vi "Process.vi"(0 "reference in":refnum<class "Logger.lvclass">, 5 "error in":errorcluster) -> (14 "reference out":refnum<class "Logger.lvclass">, 19 "error out":errorcluster)   [LabVIEW 2023, in "Logger.lvclass"]
uses:
  Logger.lvclass
  <vilib>/HPS-17000/MStream_grpc_CyclerMeasurement.ctl
  <instrlib>/HPS-17000/HPS-17000.lvclass
  <instrlib>/HPS-17000/Internal/Read Measurement Multi.vi
  Logger.lvclass/Logger.ctl
  <vilib>/Utility/SystemLogging/NI_SystemLogging.lvlib
  <vilib>/HPS-17000/NI_BC_client.lvlib
panel:
  out "error info":errorcluster
  out "Last Command":string
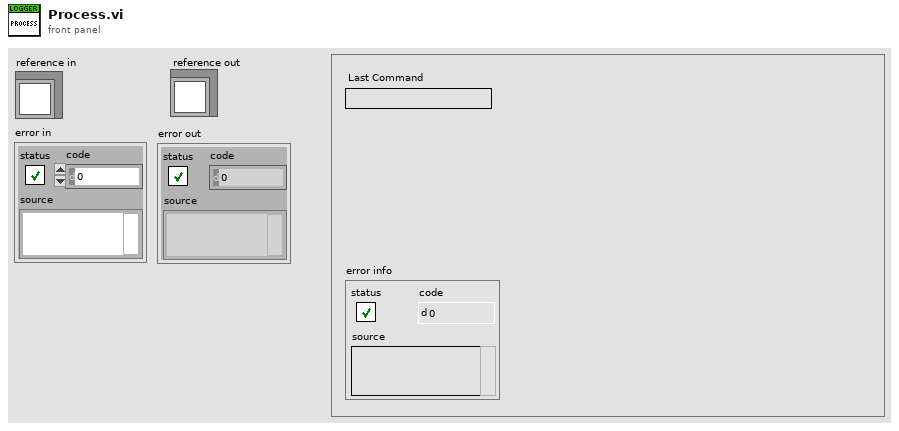
[diagram p1: front panel]
types:
  T1 = cluster{"Core":cluster{"Timeout":i32, "Events":cluster{"EventsToProcess":refnum<event-registration>}, "EventFromProcess":refnum<user-event>, "ProcessSyncQueue":refnum<queue>, "QueueFromProcess":refnum<queue>, "Command":string, "Data":variant}, "Log File Format":string, "Output Directory":path, "Log File Type":enum16{"TDMS", "CSV"}, "TDMS File":refnum<k34>, "CSV File":refnum<file>, "Logger Queue":refnum<queue>, "HPS17K Refs":refnum<class "HPS-17000.lvclass">[], "Generated Log":path, "Log Enabled":bool, "Log Created":bool}
  T2 = enum16{"open", "open or create", "create or replace", "create", "open (read-only)"}
  T3 = enum16{"open", "replace", "create", "open or create", "replace or create", "replace or create with confirmation"}
  T4 = enum32{"Invalid", "Standard", "Closed", "Hidden", "Minimized", "Maximized"}
  T5 = cluster{"EventsToProcess":refnum<event-registration>}
  T6 = typedef "Logger.lvclass/ObjectAttributes.ctl" = cluster{"Output Directory":path, "Log File Type":enum16{"TDMS", "CSV"}, "Logger Queue":refnum<queue>, "HPS17K Refs":refnum<class "HPS-17000.lvclass">[]}
  T7 = typedef "NI_BC_client.lvlib/MStream_grpc_CyclerMeasurement.ctl" = cluster{"measured_voltage":sgl, "measured_current":sgl, "setpoint_voltage":sgl, "setpoint_current":sgl, "timestamp":i64}
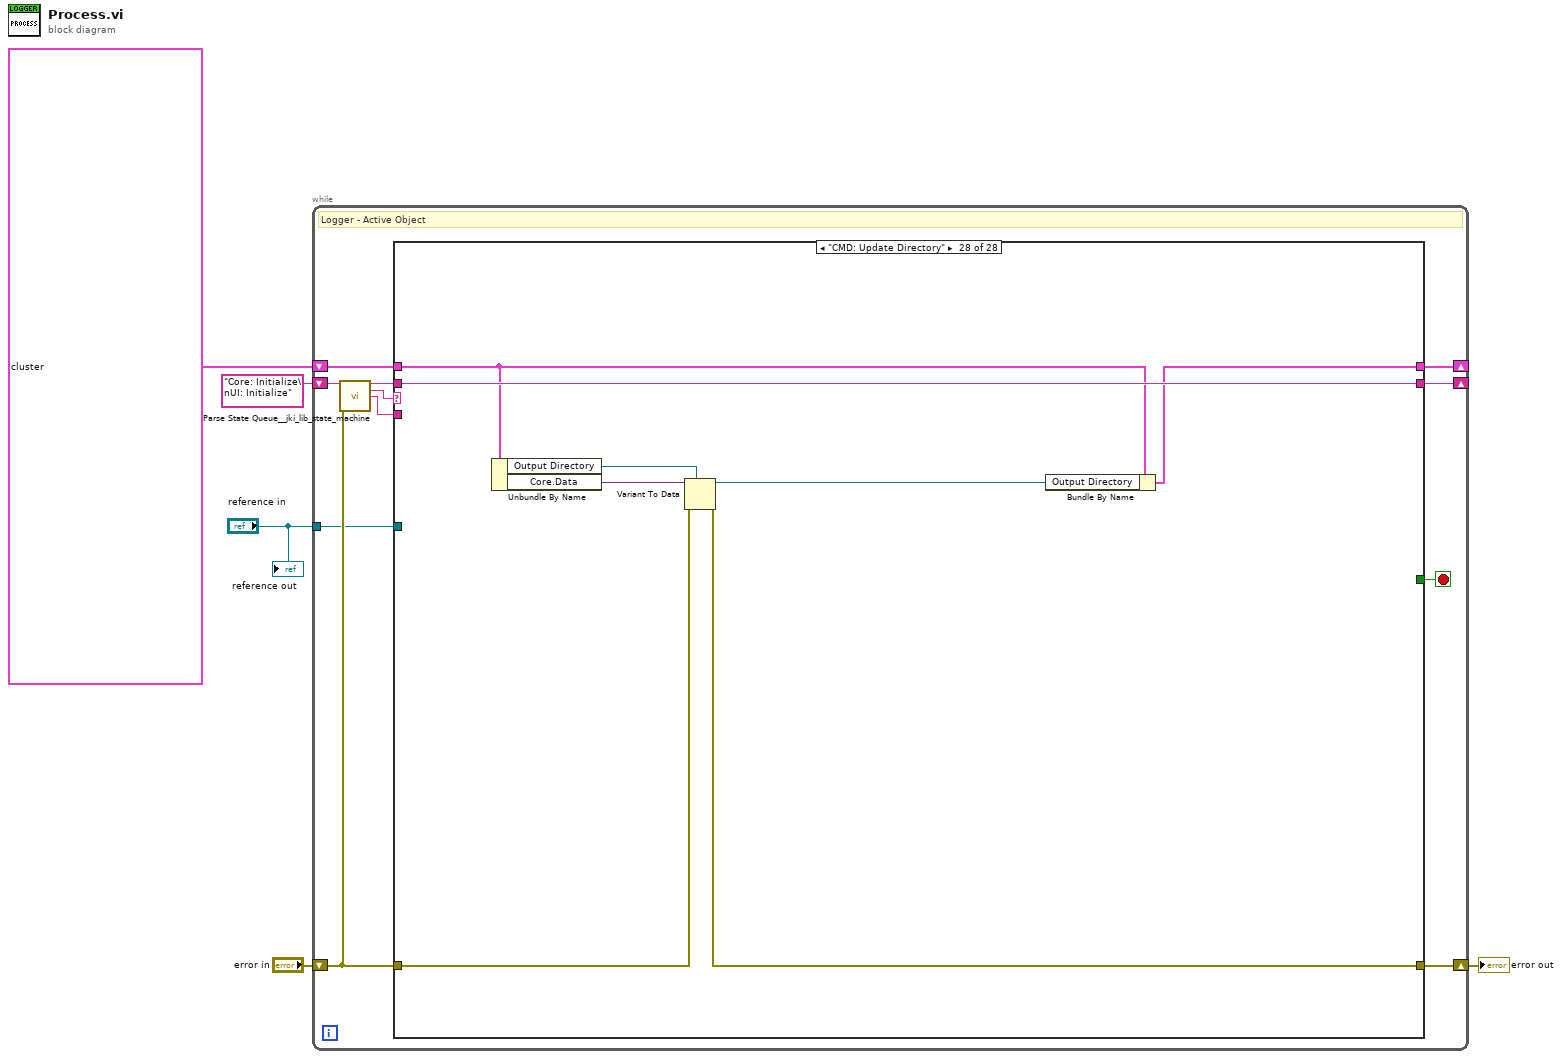
[diagram p0: block diagram]
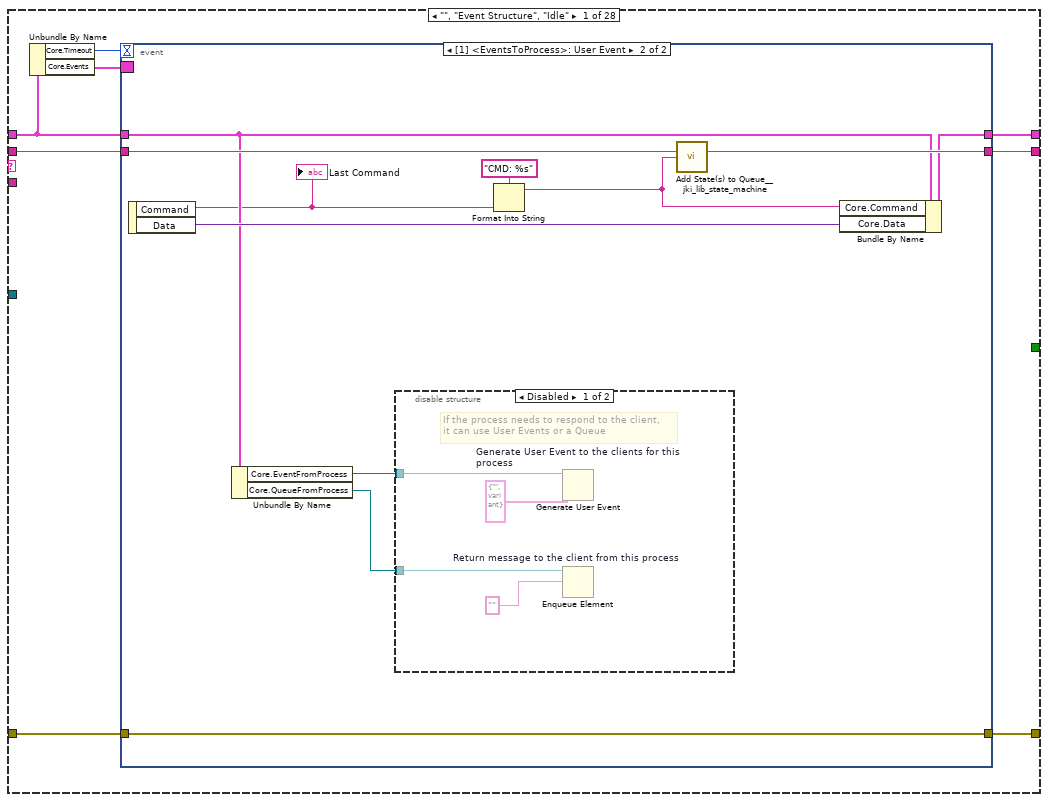
[diagram p2: hidden frame]
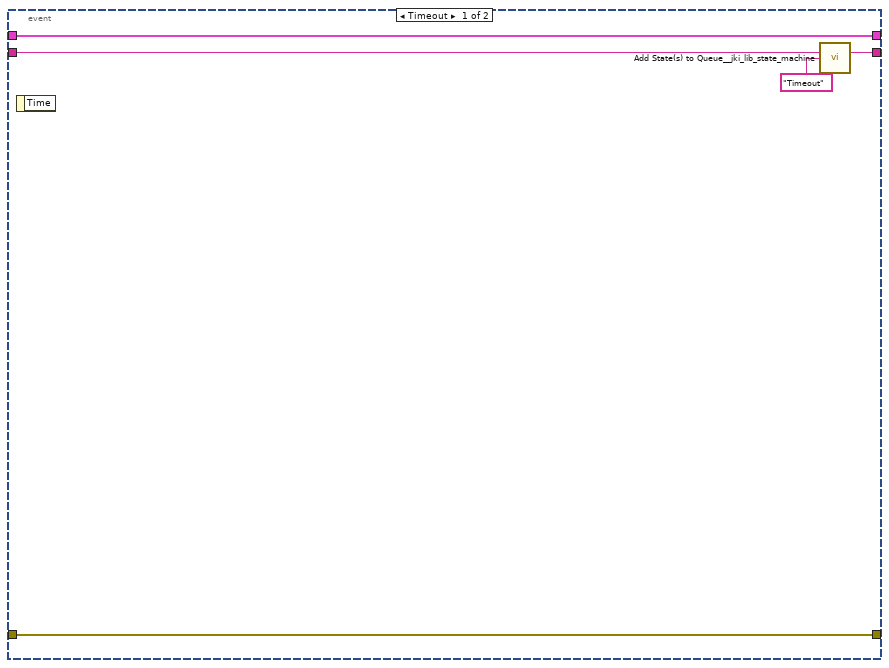
[diagram p3: hidden frame]
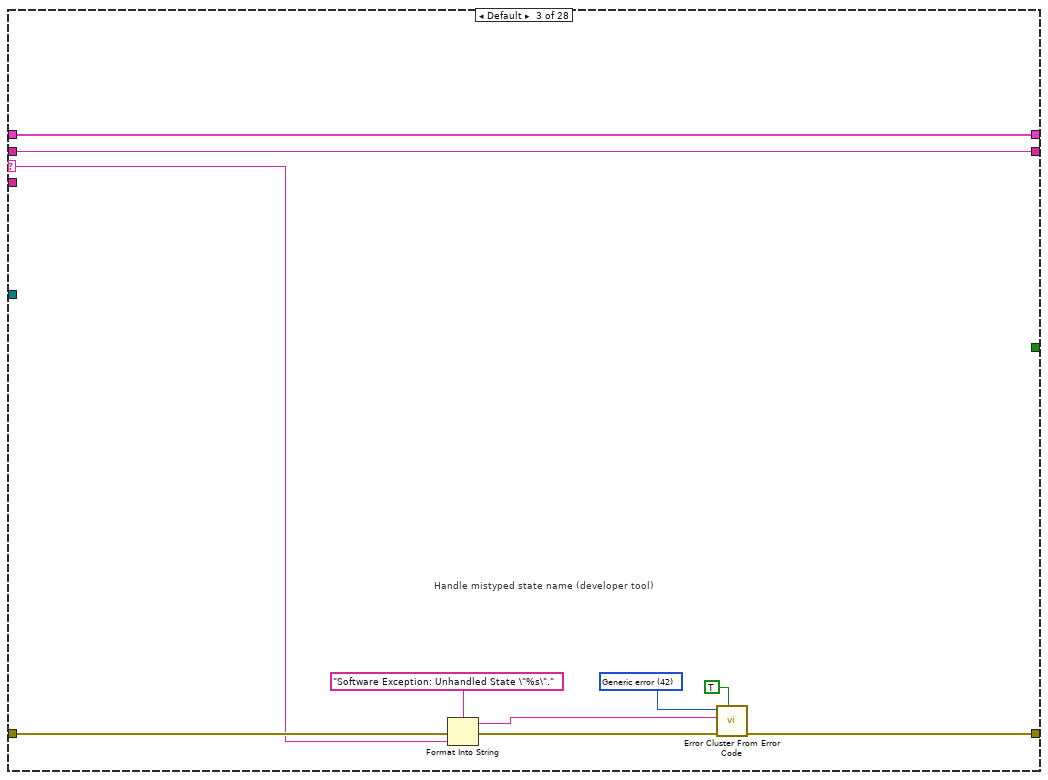
[diagram p6: hidden frame]
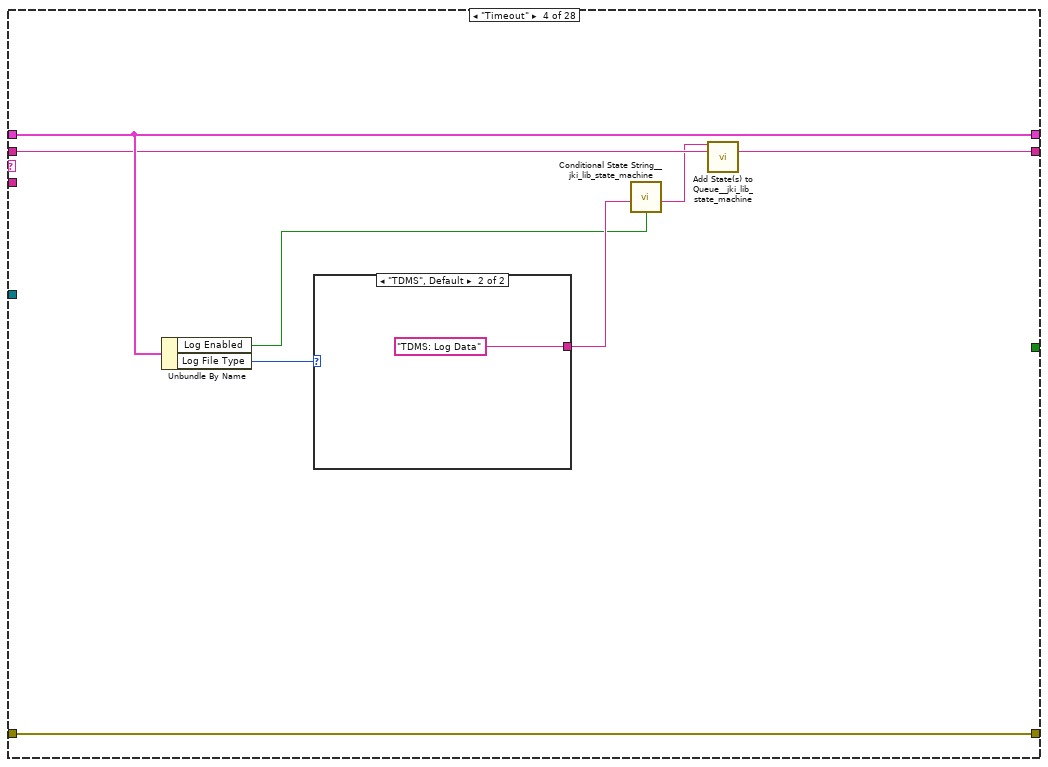
[diagram p7: hidden frame]
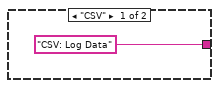
[diagram p8: hidden frame]
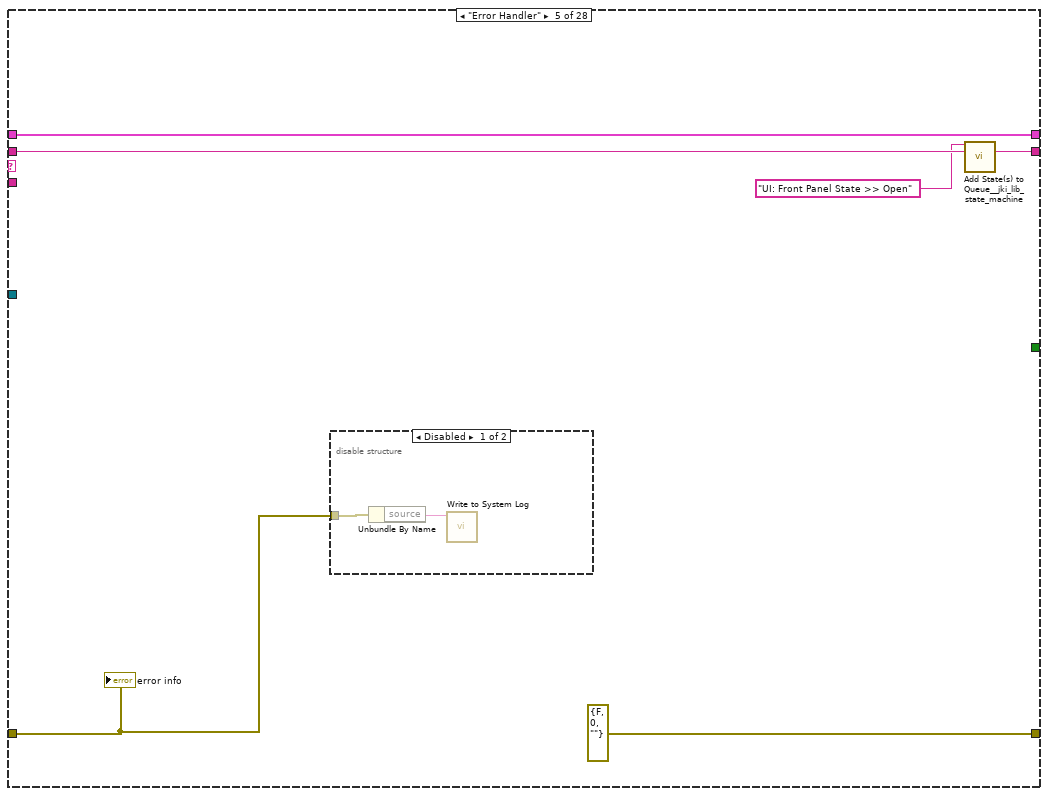
[diagram p9: hidden frame]
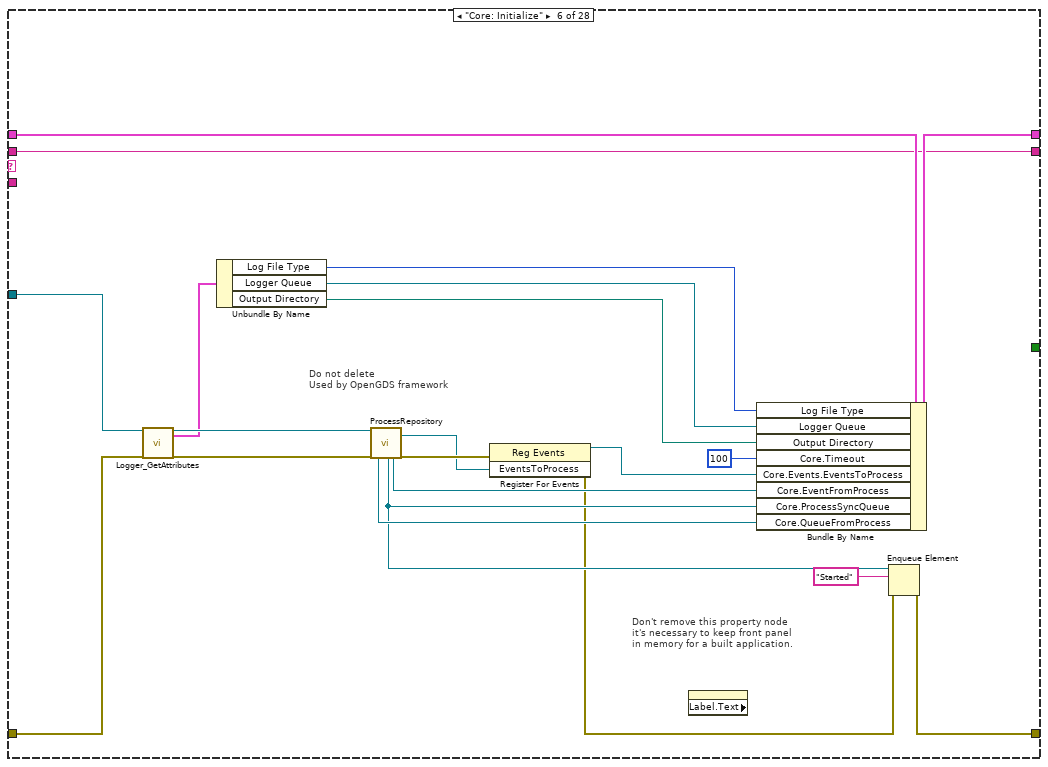
[diagram p11: hidden frame]
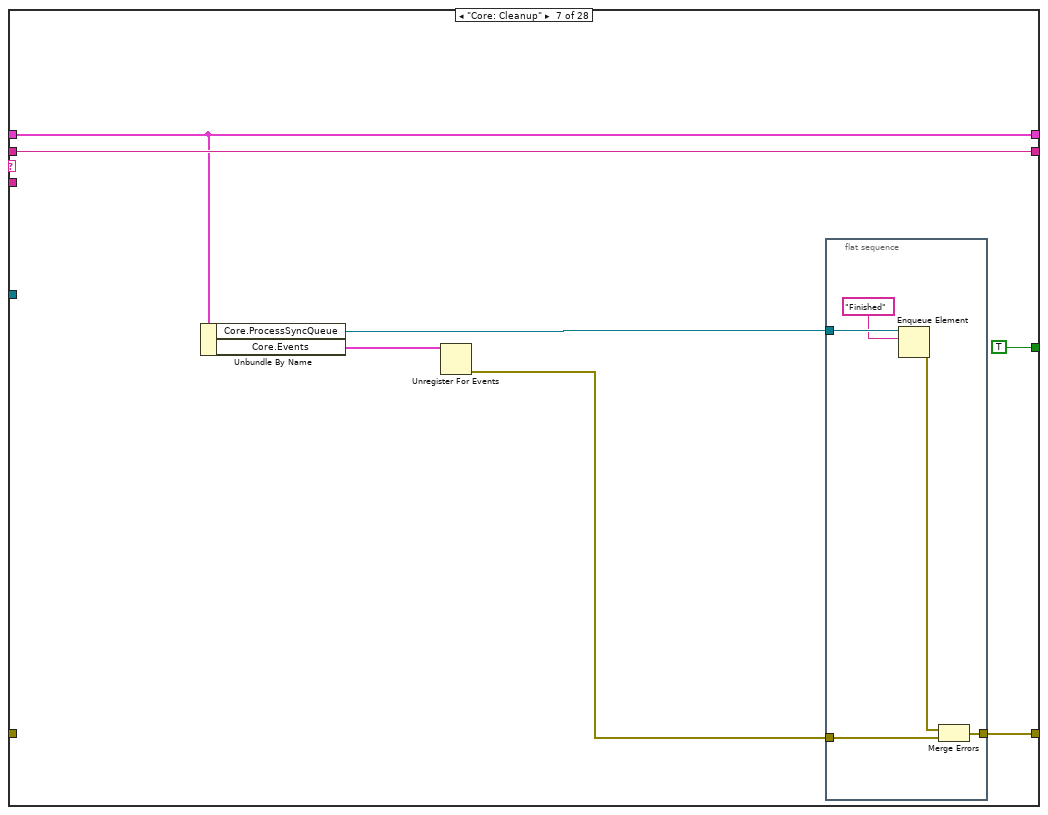
[diagram p12: hidden frame]
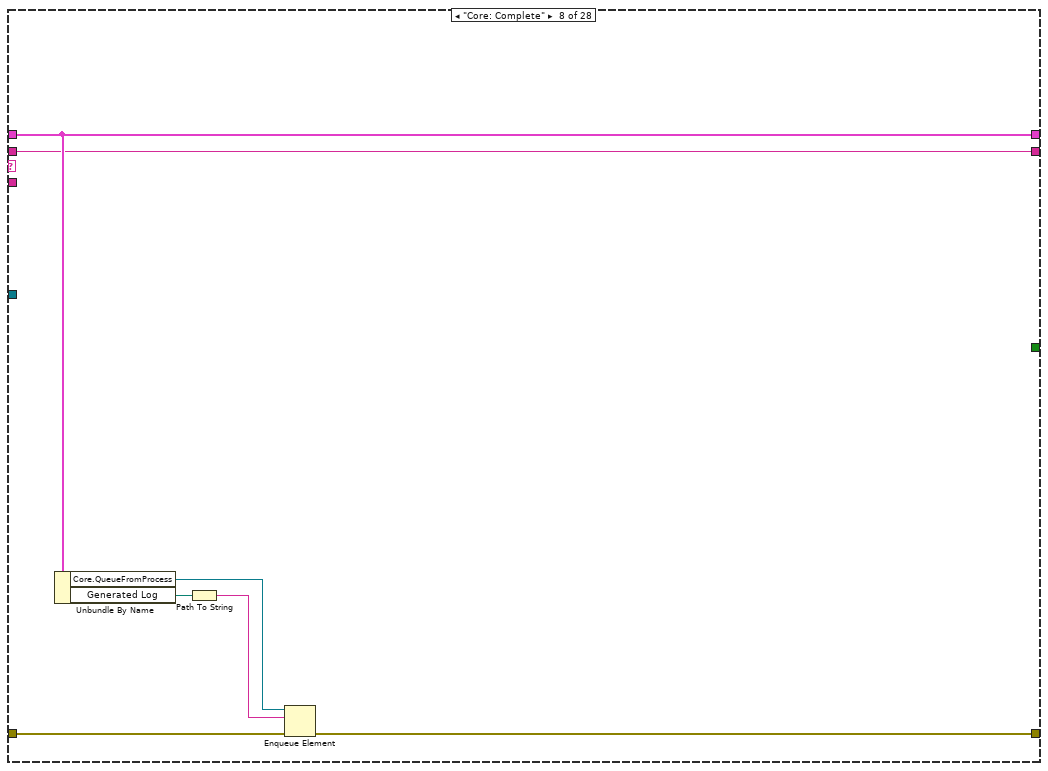
[diagram p13: hidden frame]
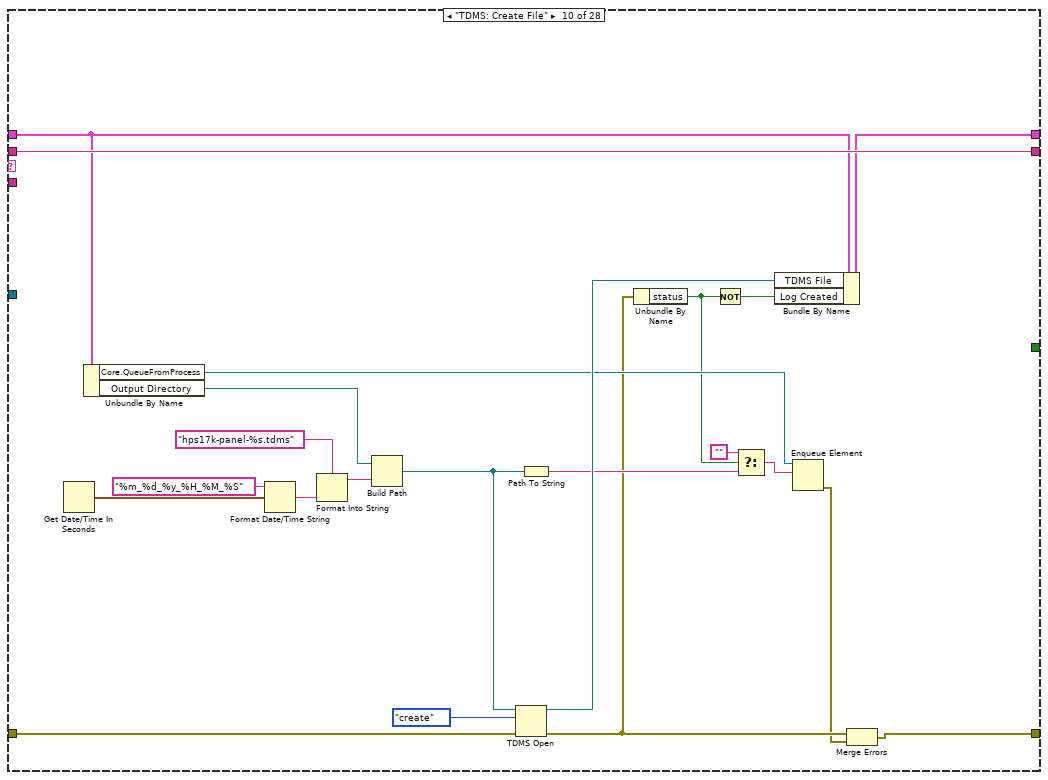
[diagram p15: hidden frame]
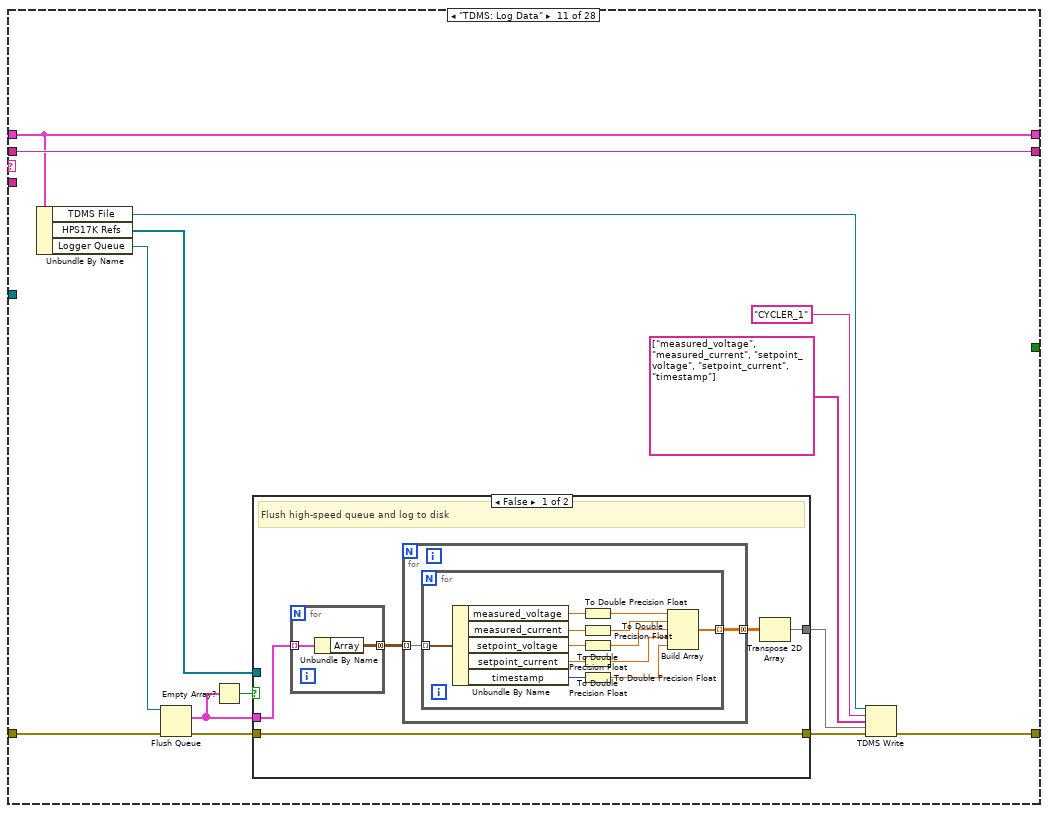
[diagram p16: hidden frame]
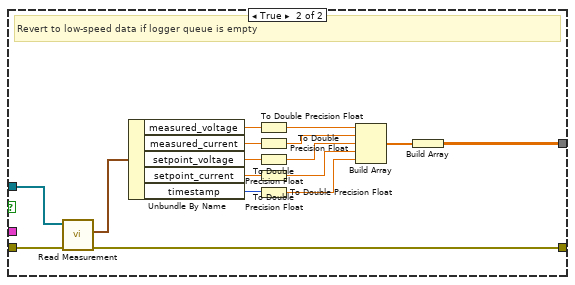
[diagram p17: hidden frame]
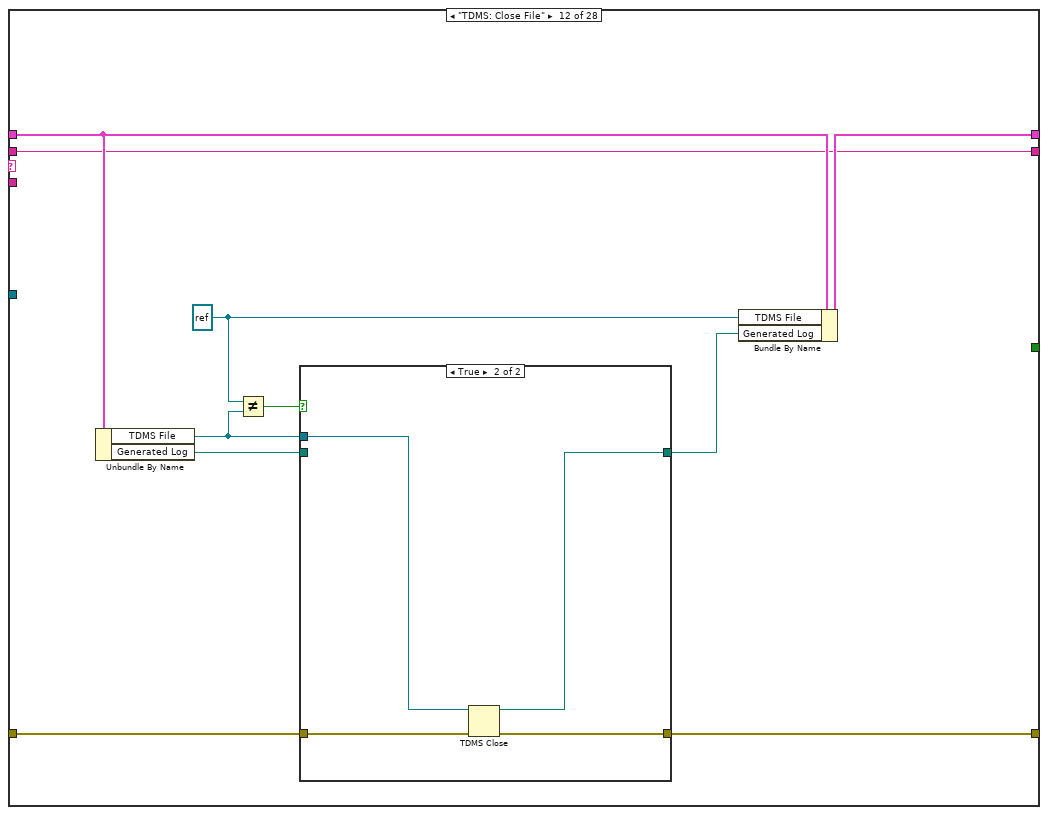
[diagram p18: hidden frame]
diagram:
  n1 = while {
    shift-right: [w15] -> w4
    shift-left: "error in" -> [w16]
    shift-right: [w8] -> _
    shift-left: "Core: Initialize\nUI: Initialize" ("States Out") -> [w11]
    shift-right: [w14] -> _
    shift-left: T1 {"Core"={"Timeout"=-1, "Events"={"EventsToProcess"=refnum}, "EventFromProcess"=refnum, "ProcessSyncQueue"=refnum, "QueueFromProcess"=refnum, "Command"="", "Data"=variant}, "Log File Format"="", "Output Directory"=path "", "Log File Type"=enum."TDMS", "TDMS File"=refnum, "CSV File"=refnum, "Logger Queue"=refnum, "HPS17K Refs"=[], "Generated Log"=path "", "Log Enabled"=FALSE, "Log Created"=FALSE} ("LocalVariables") -> [w13]
    tunnel: "reference in" -> [w6]
    stop <- w7 stop-if-true
    # "Logger - Active Object"
    n2 = call <vilib>:"Parse State Queue__jki_lib_state_machine.vi"("State Queue"=w11, "Error In (no error)"=w16) -> ("Remaining States"=w10:string, "Current State"=w12:string, "Arguments"=w9:string)  [unwired: 11 in]
    n3 = case shown="\"CMD: Update Directory\"" w12 {
      selector: w12 -> [_ _ w48 _ _ _ _ _ _ _ _ _ _ _ _ _ _ _ _ _ _ _ _ _ _ _ _ _]
      tunnel: w16 -> [w18 w47 w50 w65 w69 w82 _ w113 w118 w139 w151 w199 w210 w230 w248 w273 w277 w278 w301 _ w308 w314 w324 w332 w341 w343 w355 w358]
      tunnel: [w19 w47 w49 w65 errorcluster {"status"=FALSE, "code"=0, "source"=""} ("error constant") w96 w99 w112 w118 w119 w153 w198 w210 w218 w245 w272 w277 w278 w301 w302 w308 w314 w324 w332 w341 w342 w355 w357] -> w15
      tunnel: [w24 w46 w57 w64 w73 w95 w100 w115 w117 w137 w152 w201 w209 w227 w249 w270 w276 w280 w293 w303 w307 w313 w323 w328 w340 w349 w351 w362] -> w14
      tunnel: w13 -> [w20 w46 w57 w64 w73 w94 w100 w115 w117 w135 w152 w200 w209 w228 w249 w271 w276 w280 w293 w303 w307 w313 w323 w328 w340 w348 w352 w361]
      tunnel: w10 -> [w22 w45 w56 w62 w72 w76 w103 w111 w116 w140 w154 w192 w208 w237 w250 w267 w275 w281 w300 w305 w306 _ w320 w330 w339 w350 w354 w363]
      tunnel: w9 -> [_ _ _ _ _ _ _ _ _ _ _ _ _ _ _ _ _ w279 _ _ _ _ _ _ w336 _ _ _]
      tunnel: [w21 w45 w56 w61 w71 w76 w103 w111 w116 w140 w154 w192 w208 w237 w250 w267 w275 w281 w300 w305 w306 w310 w321 w329 w338 w350 w354 w363] -> w8
      tunnel: [_ _ _ _ _ _ TRUE _ _ _ _ _ _ _ _ _ _ _ _ _ _ _ _ _ _ _ _ _] -> w7
      tunnel: w6 -> [_ _ _ _ _ w85 _ _ _ _ _ _ _ _ _ _ _ _ _ _ _ _ _ _ _ _ _ _]
      frame "", "Event Structure", "Idle" {
        n4 = Unbundle By Name(w20) -> ("Core.Timeout"=w17:i32, "Core.Events"=w23:T5)
        n5 = event shown="[1] <EventsToProcess>: User Event" {
          selector: w23 -> [_ _]
          dyn-events: _ -> [_ _]
          timeout: w17 -> [_ _]
          tunnel: w20 -> [w29 w33]
          tunnel: [w29 w38] -> w24
          tunnel: [w27 w40] -> w21
          tunnel: w22 -> [w28 w39]
          tunnel: [w25 w34] -> w19
          tunnel: w18 -> [w25 w34]
          event Timeout {
            n6 = event-data() -> ()  [unwired: 1 in, 1 out]
            n7 = call <vilib>:"Add State(s) to Queue__jki_lib_state_machine.vi"("State(s) in (\"\")"=w28, "State(s) at Back (\"\")"="Timeout" ("State(s) at Back (\"\")")) -> ("States Out"=w27:string)  [unwired: 13 in]
          }
          event User Event {
            n8 = event-data() -> ("Command"=w31:string, "Data"=w37:variant)  [unwired: 1 in]
            "Last Command" <- w31
            n9 = Unbundle By Name(w33) -> ("Core.EventFromProcess"=w36:refnum<user-event>, "Core.QueueFromProcess"=w35:refnum<queue>)
            n10 = disable-structure shown="Disabled" {
              disable-tunnel: w36 -> [w44 _]
              disable-tunnel: w35 -> [w43 _]
              frame Disabled {
                # "If the process needs to respond to the client,\nit can use User Events or a Queue"
                n11 = Generate User Event "Generate User Event to the clients for this process"(user event=w44, event data cluster=cluster{"Command":string, "Data":variant} {"Command"="", "Data"=variant} ("event data")) -> ()  [unwired: 2 in, 2 out]
                n12 = Enqueue Element "Return message to the client from this process"(queue=w43, element="") -> ()  [unwired: 2 in, 3 out]
              }
              frame Enabled {
              }
            }
            n13 = Format Into String(format string="CMD: %s", w31) -> (resulting string=w30:string)  [unwired: 2 in, 1 out]
            n14 = call <vilib>:"Add State(s) to Queue__jki_lib_state_machine.vi"("State(s) in (\"\")"=w39, "State(s) at Back (\"\")"=w30) -> ("States Out"=w40:string)  [unwired: 13 in]
            n15 = Bundle By Name(cluster=w33, "Core.Command"=w30, "Core.Data"=w37) -> (w38:T1)
          }
        }
      }
      frame "---------- Core ----------" {
      }
      frame Default {
        w54 = 42 items=["No error", "Argument error", "Memory is full", "Out of zone", "End of file", "File already open", "Generic file I/O error", "File not found", "File permission error", "Disk is full", "Duplicate path", "Too many files open", "System feature not enabled", "Resource file not found", "Cannot add resource", "Resource not found", "Image not found", "Image memory error", "Pen does not exist", "Config type invalid", "Config token not found", "Config parse error", "Config memory error", "Bad external code format", "Bad external code offset", "External code not present", "Null window", "Destroy window error", "Null menu", "Print aborted", "Bad print record", "Print driver error", "Windows error during printing", "Memory error during printing", "Print dialog error", "Generic print error", "Invalid device refnum", "Device not found", "Device parameter error", "Device unit error", "Cannot open device", "Device call aborted", "Generic error", "Cancelled by user", "Object ID too low", "Object ID too high", "Object not in heap", "Unknown heap", "Unknown object (invalid DefProc)", "Unknown object (DefProc not in table)", "Message out of range", "Invalid (null) method", "Unknown message", "Manager call not supported", "Bad address", "Network operation in progress", "Network operation timed out", "Connection is busy", "Network attribute not supported", "Network error", "Address in use", "System out of memory", "Connection aborted", "Connection refused", "Not connected", "Already connected", "Connection closed", "Initialization error (interapplication manager)", "Bad occurrence", "Wait on unbound occurrence handler", "Occurrence queue overflow", "Datalog type conflict", "Unused", "Unrecognized type (interapplication manager)", "Memory corrupt", "Failed to make temporary DLL", "Old CIN version", "Drag socket not found", "Failed to load drop-object", "Failed to register OLE object", "Failed to release OLE object", "Format specifier type mismatch", "Unknown format specifier", "Too few format specifiers", "Too many format specifiers", "Scan failed", "Newer CIN version", "Error converting to variant", "Runtime menu error", "Password tampered", "Variant attribute not found", "Incompatible variant data type", "Event data is not available", "Event Store is not present", "Occurrence is not found", "Event Queue is not created", "Event info is not available", "Refnum passed is NULL", "Error retrieving Class GUID", "Error retrieving CoClass GUID", "Error retrieving TypeLib GUID.", "Bad built application magic bytes.", "Specific driver is different from the specific driver associated with the Logical Name.", "There is no session opened to the class driver.", "Max Error", "MAX - Error with config objects", "MAX - Error loading configuration", "MAX - Group not supported"]
        # "Handle mistyped state name (developer tool)"
        n16 = Format Into String(format string="Software Exception: Unhandled State \"%s\"." ("message"), error in=w50, w48) -> (resulting string=w53:string, error out=w52:errorcluster)  [unwired: 1 in]
        n17 = call <vilib>:"Error Cluster From Error Code.vi"("show call chain? (False)"=TRUE, "error in (no error)"=w52, "error message (\"\")"=w53, "error code (0)"=w54) -> ("error out"=w49:errorcluster)  [unwired: 5 in]
      }
      frame "Timeout" {
        n18 = Unbundle By Name(w64) -> ("Log Enabled"=w58:bool, "Log File Type"=w63:enum16{"TDMS", "CSV"})
        n19 = case shown="\"TDMS\", Default" w63 {
          tunnel: ["CSV: Log Data" ("States Out") "TDMS: Log Data" ("States Out")] -> w60
          frame "CSV" {
          }
          frame "TDMS", Default {
          }
        }
        n20 = call <vilib>:"Conditional State String__jki_lib_state_machine.vi"("Do State(s)?"=w58, "State"=w60) -> ("State Out"=w59:string)  [unwired: 7 in]
        n21 = call <vilib>:"Add State(s) to Queue__jki_lib_state_machine.vi"("State(s) in Front (\"\")"=w59, "State(s) in (\"\")"=w62) -> ("States Out"=w61:string)  [unwired: 13 in]
      }
      frame "Error Handler" {
        n22 = disable-structure shown="Disabled" {
          disable-tunnel: w69 -> [w75 _]
          frame Disabled {
            n23 = Unbundle By Name(w75) -> ("source"=w74:string)
            n24 = call <vilib>:"Write to System Log.vi"("message"=w74) -> ()  [unwired: 10 in, 1 out]
          }
          frame Enabled {
          }
        }
        n25 = call <vilib>:"Add State(s) to Queue__jki_lib_state_machine.vi"("State(s) in Front (\"\")"="UI: Front Panel State >> Open" ("State(s) at Back (\"\")"), "State(s) in (\"\")"=w72) -> ("States Out"=w71:string)  [unwired: 13 in]
        "error info" <- w69
      }
      frame "Core: Initialize" {
        # "Do not delete\nUsed by OpenGDS framework"
        # "Don't remove this property node\nit's necessary to keep front panel\nin memory for a built application."
        # "Template created by VI Technologies"
        n26 = call "Logger_GetAttributes.vi"("reference in"=w85, "Error In"=w82) -> ("reference out"=w84:refnum<class "Logger.lvclass">, "Data"=w81:T6, "Error Out"=w83:errorcluster)  [unwired: 14 in, 1 out]
        n27 = Unbundle By Name(w81) -> ("Log File Type"=w79:enum16{"TDMS", "CSV"}, "Logger Queue"=w77:refnum<queue>, "Output Directory"=w80:path)
        n28 = call "ProcessRepository.vi"("reference in"=w84, "Error In"=w83) -> ("QueueFromProcess"=w89:refnum<queue>, "ProcessSyncQueue"=w87:refnum<queue>, "EventFromProcess"=w90:refnum<user-event>, "EventsToProcess"=w92:refnum<user-event>, "Error Out"=w93:errorcluster)  [unwired: 10 in, 3 out]
        n29 = register-events(error in=w93, w92) -> (reference out=w91:refnum<event-registration>, error out=w86:errorcluster)  [unwired: 1 in]
        n30 = property on="reference in" class="LVClassControl (strict)" props=["Label", "Text"]() -> ()  [unwired: 2 in, 3 out]
        n31 = Bundle By Name(cluster=w94, "Log File Type"=w79, "Logger Queue"=w77, "Output Directory"=w80, "Core.Timeout"=100, "Core.Events.EventsToProcess"=w91, "Core.EventFromProcess"=w90, "Core.ProcessSyncQueue"=w87, "Core.QueueFromProcess"=w89) -> (w95:T1)
        n32 = Enqueue Element(queue=w87, element="Started", error in (no error)=w86) -> (error out=w96:errorcluster)  [unwired: 1 in, 2 out]
      }
      frame "Core: Cleanup" {
        n33 = Unbundle By Name(w100) -> ("Core.ProcessSyncQueue"=w101:refnum<queue>, "Core.Events"=w98:T5)
        n34 = Unregister For Events(event registration refnum=w98) -> (error out=w97:errorcluster)  [unwired: 1 in]
        n35 = flat-sequence {
          tunnel: [w107] -> w99
          tunnel: w101 -> [w106]
          tunnel: w97 -> [w105]
          frame #0 {
            n36 = Enqueue Element(queue=w106, element="Finished") -> (error out=w108:errorcluster)  [unwired: 2 in, 2 out]
            n37 = Merge Errors(w108, w105) -> (w107:errorcluster)
          }
        }
      }
      frame "Core: Complete" {
        n38 = Unbundle By Name(w115) -> ("Core.QueueFromProcess"=w114:refnum<queue>, "Generated Log"=w110:path)
        n39 = Path To String(path=w110) -> (string=w109:string)
        n40 = Enqueue Element ("Return message to the client from this process")(queue=w114, element=w109, error in (no error)=w113) -> (error out=w112:errorcluster)  [unwired: 1 in, 2 out]
      }
      frame "---------- TDMS ----------" {
      }
      frame "TDMS: Create File" {
        n41 = Get Date/Time In Seconds() -> (seconds since 1Jan1904=w131:timestamp)
        n42 = Unbundle By Name(w135) -> ("Core.QueueFromProcess"=w126:refnum<queue>, "Output Directory"=w133:path)
        n43 = Format Date/Time String(time format string (%c)="%m_%d_%y_%H_%M_%S", seconds (now)=w131) -> (date/time string=w130:string)  [unwired: 1 in]
        n44 = Format Into String(format string="hps17k-panel-%s.tdms", w130) -> (resulting string=w132:string)  [unwired: 2 in, 1 out]
        n45 = Build Path(base path=w133, name or relative path=w132) -> (appended path=w127:path)
        n46 = TDMS Open(8:w139, 10:T2."create" ("operation (0:open)"), 11:w127) -> (0:w121:errorcluster, 3:w136:refnum<k34>)  [unwired: 4 in]
        n47 = Path To String(path=w127) -> (string=w123:string)
        n48 = Unbundle By Name(w121) -> ("status"=w124:bool)
        n49 = Not(x=w124) -> (.not. x?=w128:bool)
        n50 = Select(t="", s=w124, f=w123) -> (s? t:f=w122:string)
        n51 = Bundle By Name(cluster=w135, "TDMS File"=w136, "Log Created"=w128) -> (w137:T1)
        n52 = Enqueue Element(queue=w126, element=w122) -> (error out=w120:errorcluster)  [unwired: 2 in, 2 out]
        n53 = Merge Errors(w121, w120) -> (w119:errorcluster)
      }
      frame "TDMS: Log Data" {
        n54 = Unbundle By Name(w152) -> ("TDMS File"=w150:refnum<k34>, "HPS17K Refs"=w144:refnum<class "HPS-17000.lvclass">[], "Logger Queue"=w147:refnum<queue>)
        n55 = Flush Queue(queue=w147, error in (no error)=w151) -> (remaining elements=w145:cluster{"Array":T7[][]}[], error out=w143:errorcluster)  [unwired: 1 out]
        n56 = Empty Array?(array=w145) -> (empty?=w146:bool)
        n57 = case shown="False" w146 {
          tunnel: w145 -> [w157 _]
          tunnel: w144 -> [_ w190]
          tunnel: w143 -> [w155 w191]
          tunnel: [w155 w189] -> w142
          tunnel: [w158 w184] -> w141
          frame False {
            # "Flush high-speed queue and log to disk"
            n58 = for {
              tunnel: w157 -> [w161] mode=indexing
              tunnel: [w160] -> w156 mode=concatenating
              n59 = Unbundle By Name(w161) -> ("Array"=w160:T7[][])
            }
            n60 = for {
              tunnel: [w163] -> w159 mode=concatenating
              tunnel: w156 -> [w162] mode=indexing
              n61 = for {
                tunnel: w162 -> [w175] mode=indexing
                tunnel: [w172] -> w163 mode=indexing
                # "Iterate each measurement for the cycler"
                n62 = Unbundle By Name(w175) -> ("measured_voltage"=w165:sgl, "measured_current"=w167:sgl, "setpoint_voltage"=w169:sgl, "setpoint_current"=w171:sgl, "timestamp"=w174:i64)
                n63 = To Double Precision Float(number=w165) -> (double precision float=w164:dbl)
                n64 = To Double Precision Float(number=w167) -> (double precision float=w166:dbl)
                n65 = To Double Precision Float(number=w169) -> (double precision float=w168:dbl)
                n66 = To Double Precision Float(number=w171) -> (double precision float=w170:dbl)
                n67 = To Double Precision Float(number=w174) -> (double precision float=w173:dbl)
                n68 = Build Array(w164, w166, w168, w170, w173) -> (w172:dbl[])
              }
            }
            n69 = Transpose 2D Array(2D array=w159) -> (transposed array=w158:dbl[][])
          }
          frame True {
            # "Revert to low-speed data if logger queue is empty"
            n70 = call-poly <instrlib>:"Read Measurement.vi"("error in"=w191, "cycler refs in"=w190) -> ("error out"=w189:errorcluster, "aggregated cycler measurements"=w186:T7)  [unwired: 7 in, 1 out]
            n71 = Unbundle By Name(w186) -> ("measured_voltage"=w183:sgl, "measured_current"=w182:sgl, "setpoint_voltage"=w181:sgl, "setpoint_current"=w180:sgl, "timestamp"=w187:i64)
            n72 = To Double Precision Float(number=w183) -> (double precision float=w176:dbl)
            n73 = To Double Precision Float(number=w182) -> (double precision float=w177:dbl)
            n74 = To Double Precision Float(number=w181) -> (double precision float=w178:dbl)
            n75 = To Double Precision Float(number=w180) -> (double precision float=w179:dbl)
            n76 = To Double Precision Float(number=w187) -> (double precision float=w188:dbl)
            n77 = Build Array(w176, w177, w178, w179, w188) -> (w185:dbl[])
            n78 = Build Array(w185) -> (w184:dbl[][])
          }
        }
        n79 = TDMS Write(0:w150, 5:"CYCLER_1" ("group name in (Untitled)"), 7:string[] ["measured_voltage", "measured_current", "setpoint_voltage", "setpoint_current", "timestamp"] ("channel name(s) in (Untitled)"), 9:w141, 11:w142) -> (15:w153:errorcluster)  [unwired: 1 in, 3 out]
      }
      frame "TDMS: Close File" {
        w196 = refnum<k34> refnum ("TDMS File")
        n80 = Unbundle By Name(w200) -> ("TDMS File"=w197:refnum<k34>, "Generated Log"=w194:path)
        n81 = Not Equal?(x=w196, y=w197) -> (x != y?=w195:bool)
        n82 = case shown="True" w195 {
          tunnel: w199 -> [w203 w207]
          tunnel: [w203 w206] -> w198
          tunnel: w197 -> [_ w205]
          tunnel: w194 -> [w202 _]
          tunnel: [w202 w204] -> w193
          frame False {
          }
          frame True {
            n83 = TDMS Close(8:w207, 11:w205) -> (0:w206:errorcluster, 3:w204:path)
          }
        }
        n84 = Bundle By Name(cluster=w200, "TDMS File"=w196, "Generated Log"=w193) -> (w201:T1)
      }
      frame "---------- CSV ----------" {
      }
      frame "CSV: Create File" {
        n85 = Get Date/Time In Seconds() -> (seconds since 1Jan1904=w234:timestamp)
        n86 = Unbundle By Name(w228) -> ("Core.QueueFromProcess"=w212:refnum<queue>, "Output Directory"=w231:path)
        n87 = Format Date/Time String(time format string (%c)="%m_%d_%y_%H_%M_%S", seconds (now)=w234) -> (date/time string=w233:string)  [unwired: 1 in]
        n88 = Format Into String(format string="hps17k-panel-%s.csv", w233) -> (resulting string=w235:string)  [unwired: 2 in, 1 out]
        n89 = Build Path(base path=w231, name or relative path=w235) -> (appended path=w216:path)
        n90 = Open/Create/Replace File(file path (use dialog)=w216, error in=w230, operation (0:open)=T3."create") -> (refnum out=w226:refnum<file>, error out=w225:errorcluster)  [unwired: 3 in, 1 out]
        n91 = Array To Spreadsheet String(delimiter (Tab)=",", array=string[] ["measured_voltage", "measured_current", "setpoint_voltage", "setpoint_current", "timestamp_ns"] ("channel name(s) in (Untitled)"), 3:"%s" ("format string")) -> (spreadsheet string=w221:string)
        n92 = Write to Text File(file (use dialog)=w226, text=w221, error in=w225) -> (refnum out=w217:refnum<file>, error out=w219:errorcluster)  [unwired: 1 in, 1 out]
        n93 = Unbundle By Name(w219) -> ("status"=w214:bool)
        n94 = Path To String(path=w216) -> (string=w215:string)
        n95 = Not(x=w214) -> (.not. x?=w220:bool)
        n96 = Select(t="", s=w214, f=w215) -> (s? t:f=w213:string)
        n97 = Bundle By Name(cluster=w228, "CSV File"=w217, "Log Created"=w220) -> (w227:T1)
        n98 = Enqueue Element(queue=w212, element=w213, error in (no error)=w219) -> (error out=w218:errorcluster)  [unwired: 1 in, 2 out]
      }
      frame "CSV: Log Data" {
        n99 = Unbundle By Name(w249) -> ("CSV File"=w244:refnum<file>, "Logger Queue"=w247:refnum<queue>)
        n100 = Flush Queue(queue=w247, error in (no error)=w248) -> (remaining elements=w240:cluster{"Array":T7[][]}[], error out=w246:errorcluster)  [unwired: 1 out]
        n101 = for {
          tunnel: w240 -> [w266] mode=indexing
          tunnel: [w265] -> w239 mode=concatenating
          n102 = Unbundle By Name(w266) -> ("Array"=w265:T7[][])
        }
        n103 = for {
          tunnel: w239 -> [w252] mode=indexing
          tunnel: [w251] -> w238 mode=concatenating
          # "Iterate each group of cycler data"
          n104 = for {
            tunnel: w252 -> [w264] mode=indexing
            tunnel: [w263] -> w251 mode=indexing
            # "Iterate each measurement for the cycler"
            n105 = Unbundle By Name(w264) -> ("measured_voltage"=w262:sgl, "measured_current"=w261:sgl, "setpoint_voltage"=w260:sgl, "setpoint_current"=w259:sgl, "timestamp"=w258:i64)
            n106 = To Double Precision Float(number=w262) -> (double precision float=w257:dbl)
            n107 = To Double Precision Float(number=w261) -> (double precision float=w256:dbl)
            n108 = To Double Precision Float(number=w260) -> (double precision float=w255:dbl)
            n109 = To Double Precision Float(number=w259) -> (double precision float=w254:dbl)
            n110 = To Double Precision Float(number=w258) -> (double precision float=w253:dbl)
            n111 = Build Array(w257, w256, w255, w254, w253) -> (w263:dbl[])
          }
        }
        n112 = Array To Spreadsheet String(delimiter (Tab)=",", array=w238, 3:"%f" ("format string")) -> (spreadsheet string=w241:string)
        n113 = Write to Text File(file (use dialog)=w244, text=w241, error in=w246) -> (error out=w245:errorcluster)  [unwired: 1 in, 2 out]
      }
      frame "CSV: Close File" {
        n114 = Unbundle By Name(w271) -> ("CSV File"=w274:refnum<file>)
        n115 = Close File(refnum=w274, error in=w273) -> (path=w268:path, error out=w272:errorcluster)
        n116 = Bundle By Name(cluster=w271, "CSV File"=refnum<file> refnum, "Generated Log"=w268) -> (w270:T1)
      }
      frame "---------- UI ----------" {
      }
      frame "UI: Front Panel State" {
        n117 = case shown="\"Close\"" w279 {
          frame "Open", Default {
            n118 = property class="VI"() -> ("FP.State"=w282:T4)  [unwired: 2 in, 2 out]
            n119 = case shown="Default" w282 {
              frame Default {
                n120 = invoke class="VI" method="FP.Open"("Activate"=TRUE, "State"=T4."Standard") -> ()  [unwired: 3 in, 5 out]
              }
              frame "Standard" {
              }
            }
          }
          frame "Close" {
            n121 = property class="VI"() -> ("FP.State"=w285:T4)  [unwired: 2 in, 2 out]
            n122 = case shown="Default" w285 {
              frame "Closed" {
              }
              frame Default {
                n123 = invoke class="VI" method="FP.Close"() -> ()  [unwired: 3 in, 3 out]
              }
            }
          }
        }
      }
      frame "UI: Initialize" {
        n124 = property class="VI"() -> ("Name"=w299:string)  [unwired: 2 in, 2 out]
        n125 = Match Pattern(string=w299, regular expression="\\2Evi$") -> (before substring=w297:string)  [unwired: 1 in, 3 out]
        n126 = Reverse String(1:w297) -> (0:w296:string)
        n127 = Match Pattern(string=w296, regular expression=":") -> (before substring=w294:string, after substring=w292:string)  [unwired: 1 in, 2 out]
        n128 = Match Pattern(string=w292, regular expression="\\2E") -> (after substring=w290:string)  [unwired: 1 in, 3 out]
        n129 = Reverse String(1:w290) -> (0:w289:string)
        n130 = Reverse String(1:w294) -> (0:w288:string)
        n131 = Format Into String(format string="%s %s", w289, w288) -> (resulting string=w287:string)  [unwired: 2 in, 1 out]
        n132 = property class="VI"("Front Panel.Title"=w287) -> ()  [unwired: 2 in, 2 out]
      }
      frame "UI: Cleanup" {
        n133 = property class="VI"() -> (error out=w302:errorcluster, "FP.State"=w304:T4)  [unwired: 2 in, 1 out]
        n134 = case shown="\"Standard\", Default" w304 {
          frame "Closed" {
          }
          frame "Standard", Default {
            n135 = invoke class="VI" method="FP.Close"() -> ()  [unwired: 3 in, 3 out]
          }
        }
      }
      frame "---------- CMD ----------" {
      }
      frame "CMD: Exit" {
        n136 = Unbundle By Name(w313) -> ("Log File Type"=w312:enum16{"TDMS", "CSV"})
        n137 = case shown="\"TDMS\", Default" w312 {
          tunnel: ["TDMS: Close File" ("State(s) in Front (\"\")") "CSV: Close File" ("State(s) in Front (\"\")")] -> w309
          frame "TDMS", Default {
          }
          frame "CSV" {
          }
        }
        n138 = call <vilib>:"Add State(s) to Queue__jki_lib_state_machine.vi"("State(s) in Front (\"\")"=w309, "State(s) in (\"\")"="UI: Cleanup\nCore: Cleanup" ("State(s) at Back (\"\")")) -> ("States Out"=w310:string)  [unwired: 13 in]
      }
      frame "CMD: Close Log" {
        n139 = Unbundle By Name(w323) -> ("Log File Type"=w322:enum16{"TDMS", "CSV"})
        n140 = case shown="\"CSV\"" w322 {
          tunnel: ["TDMS: Close File" ("State(s) in Front (\"\")") "CSV: Close File" ("State(s) in Front (\"\")")] -> w319
          frame "TDMS", Default {
          }
          frame "CSV" {
          }
        }
        n141 = call <vilib>:"Add State(s) to Queue__jki_lib_state_machine.vi"("State(s) in (\"\")"=w319, "State(s) at Back (\"\")"="Core: Complete" ("State(s) at Back (\"\")")) -> ("States Out"=w318:string)  [unwired: 13 in]
        n142 = call <vilib>:"Add State(s) to Queue__jki_lib_state_machine.vi"("State(s) in Front (\"\")"=w318, "State(s) in (\"\")"=w320) -> ("States Out"=w321:string)  [unwired: 13 in]
      }
      frame "CMD: Create Log" {
        n143 = Unbundle By Name(w328) -> ("Log File Type"=w327:enum16{"TDMS", "CSV"})
        n144 = case shown="\"TDMS\", Default" w327 {
          tunnel: ["TDMS: Create File" ("States Out") "CSV: Create File" ("States Out")] -> w331
          frame "TDMS", Default {
          }
          frame "CSV" {
          }
        }
        n145 = call <vilib>:"Add State(s) to Queue__jki_lib_state_machine.vi"("State(s) in Front (\"\")"=w331, "State(s) in (\"\")"=w330) -> ("States Out"=w329:string)  [unwired: 13 in]
      }
      frame "CMD: Front Panel State" {
        n146 = Format Into String(format string="UI: Front Panel State>>%s" ("string"), w336) -> (resulting string=w335:string)  [unwired: 2 in, 1 out]
        n147 = call <vilib>:"Add State(s) to Queue__jki_lib_state_machine.vi"("State(s) in (\"\")"=w339, "State(s) at Back (\"\")"=w335) -> ("States Out"=w338:string)  [unwired: 13 in]
      }
      frame "CMD: Start Log" {
        n148 = Unbundle By Name(w348) -> ("Log Created"=w346:bool, "Logger Queue"=w344:refnum<queue>)
        n149 = Flush Queue(queue=w344, error in (no error)=w343) -> (error out=w342:errorcluster)  [unwired: 2 out]
        n150 = And(x=TRUE ("Enable"), y=w346) -> (x .and. y?=w345:bool)
        n151 = Bundle By Name(cluster=w348, "Log Enabled"=w345) -> (w349:T1)
      }
      frame "CMD: Stop Log" {
        n152 = Bundle By Name(cluster=w352, "Log Enabled"=FALSE ("Enable")) -> (w351:T1)
      }
      frame "CMD: Update Directory" {
        n153 = Unbundle By Name(w361) -> ("Output Directory"=w360:path, "Core.Data"=w359:variant)
        n154 = Variant To Data(error in=w358, type=w360, Variant=w359) -> (data=w356:path, error out=w357:errorcluster)
        n155 = Bundle By Name(cluster=w361, "Output Directory"=w356) -> (w362:T1)
      }
    }
  }
  "error out" <- w4
  "reference out" <- "reference in"
